vi "Aliases Page.vi"(8 "error in (no error)":errorcluster, 11 "Node Ptr":T4 format="%.0x") -> (0 "error out":errorcluster)   [LabVIEW 2017, in "Routing and Faulting System Explorer.lvlib"]
uses:
  Routing and Faulting System Explorer.lvlib
  <vilib>/NI Veristand/Custom Device API/Custom Device Item Ref.ctl
  Alias.ctl
  Endpoint.ctl
  Shared/UI Common/Sort Button.ctl
  Aliases Page Controls.ctl
  16100924-b29d-4153-bcd0-e39b01036c8d.vi
  16100924-b29d-4153-bcd0-e39b01036c8d.vi/8c7ce3ae-3804-454d-a5c4-51ab498be0b3.vi
  16100924-b29d-4153-bcd0-e39b01036c8d.vi/30b866c3-8f47-4b43-8d37-8753fc540d9b.vi
  <vilib>/NI VeriStand/Custom Device API/Custom Device API.lvlib
  Shared/UI Common/UI Common.lvlib
panel:
  in  "Sort":T1
  out "Alias":string="Alias"
  out "Endpoint":string="Endpoint"
  out "Aliases":T2[](array[typedef])
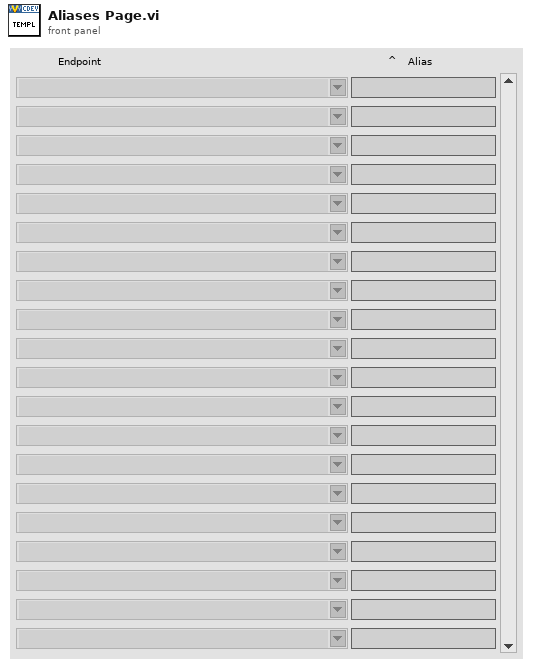
[diagram p1: front panel]
types:
  T1 = typedef "UI Common.lvlib/Sort Button.ctl" = bool
  T2 = typedef "Routing and Faulting System Explorer.lvlib/Alias.ctl" = cluster{"Endpoint":T3, "Alias":string}
  T3 = typedef "Routing and Faulting System Explorer.lvlib/Endpoint.ctl" = string
  T4 = typedef "Custom Device API.lvlib/Custom Device Item Ref.ctl" = u64
  T5 = typedef "Routing and Faulting System Explorer.lvlib/Aliases Page Controls.ctl" = cluster{"Aliases":refnum<vi>, "Endpoint":refnum<vi>, "Alias":refnum<vi>, "Sort":refnum<vi>}
  T6 = typedef "Custom Device API.lvlib/Custom Device Commands.ctl" = enum16{"Default", "Item renamed", "Shutdown", "Dynamic button pressed"}
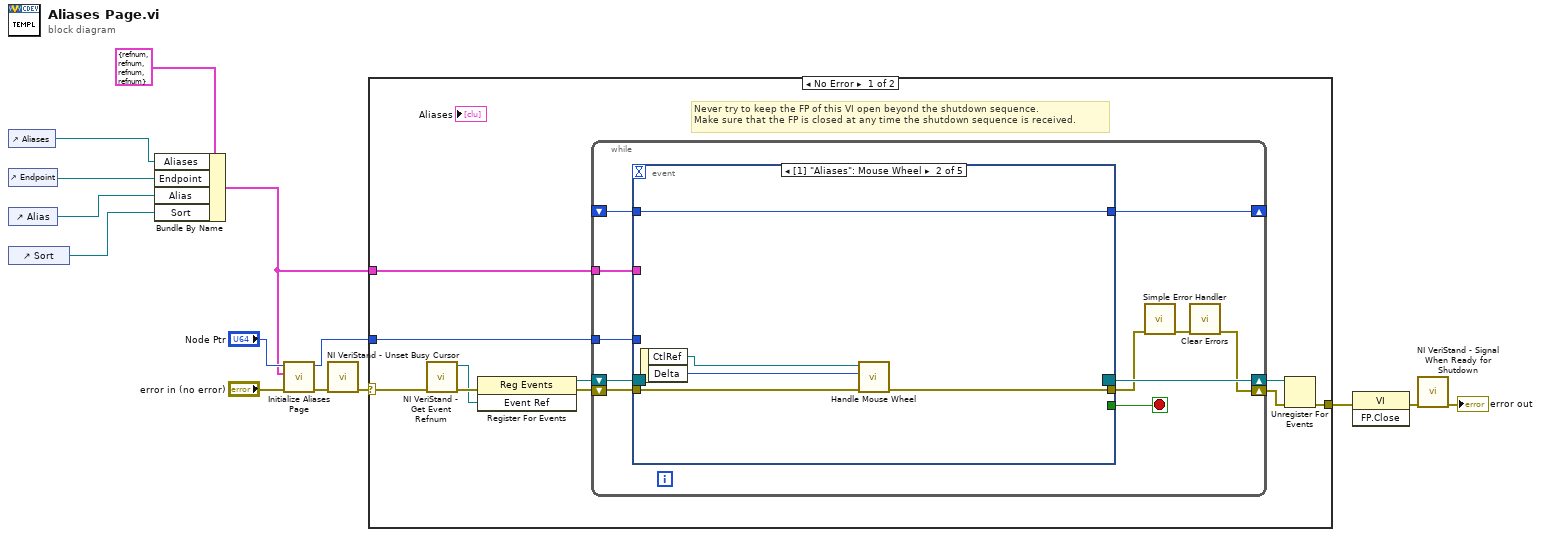
[diagram p0: block diagram]
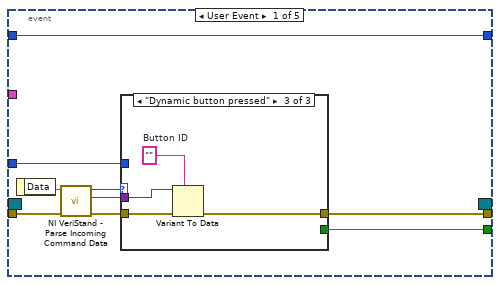
[diagram p2: hidden frame]
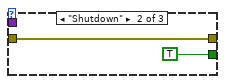
[diagram p4: hidden frame]
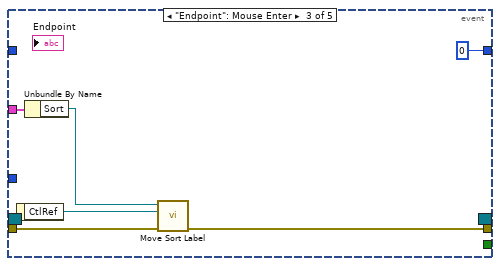
[diagram p5: hidden frame]
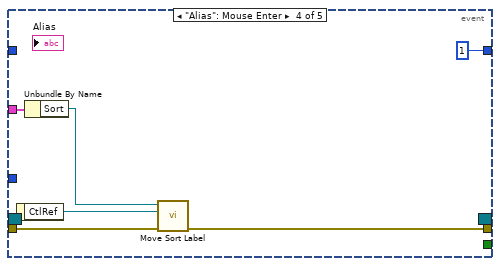
[diagram p6: hidden frame]
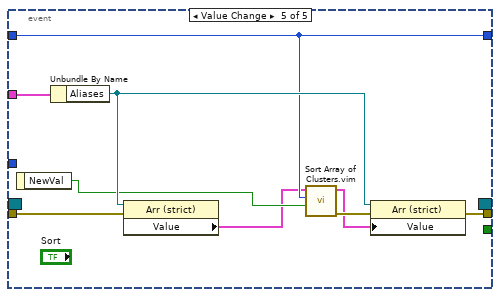
[diagram p7: hidden frame]
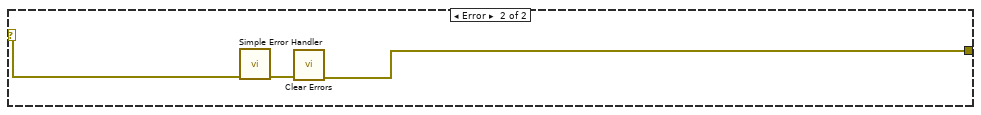
[diagram p8: hidden frame]
diagram:
  n1 = control-ref of="Aliases"() -> (w1:refnum<vi>)
  n2 = control-ref of="Endpoint"() -> (w8:refnum<vi>)
  n3 = control-ref of="Alias"() -> (w7:refnum<vi>)
  n4 = control-ref of="Sort"() -> (w6:refnum<vi>)
  n5 = Bundle By Name(cluster=T5 {"Aliases"=refnum, "Endpoint"=refnum, "Alias"=refnum, "Sort"=refnum} ("Aliases Page Controls"), "Aliases"=w1, "Endpoint"=w8, "Alias"=w7, "Sort"=w6) -> (w2:T5)
  n6 = call "Initialize Aliases Page.vi"("error in (no error)"="error in (no error)", "Aliases Page Controls"=w2, "Aliases Ref in"="Node Ptr") -> ("error out"=w5:errorcluster, "Aliases Ref out"=w9:T4)  [unwired: 7 in]
  n7 = call <vilib>:"NI VeriStand - Unset Busy Cursor.vi"("error in (no error)"=w5) -> ("error out"=w12:errorcluster)  [unwired: 10 out]
  n8 = case shown="No Error" w12 {
    selector: w12 -> [w19 w80]
    tunnel: [w22 w78] -> w14
    tunnel: w9 -> [w20 _]
    tunnel: w2 -> [w17 _]
    frame No Error {
      # "Never try to keep the FP of this VI open beyond the shutdown sequence.\nMake sure that the FP is closed at any time the shutdown sequence is received."
      n9 = call <vilib>:"NI VeriStand - Get Event Refnum.vi"("error in (no error)"=w19) -> ("error out"=w16:errorcluster, "Event Ref"=w15:refnum<user-event>)  [unwired: 9 out]
      n10 = register-events(error in=w16, w15) -> (reference out=w21:refnum<event-registration>, error out=w18:errorcluster)  [unwired: 1 in]
      n11 = while {
        tunnel: w20 -> [w31]
        shift-right: [w28] -> w23
        shift-left: w18 -> [w34]
        shift-right: [w35] -> w24
        shift-left: w21 -> [w33]
        shift-right: [w27] -> _
        shift-left: _ -> [w25]
        tunnel: w17 -> [w26]
        stop <- w32 stop-if-true
        n12 = event shown="[1] \"Aliases\": Mouse Wheel" {
          selector: w33 -> [_ _ _ _ _]
          dyn-events: [_ _ _ _ _] -> w35
          timeout: _ -> [_ _ _ _ _]
          tunnel: w34 -> [w44 w54 w62 w68 w77]
          tunnel: [w40 _ _ _ _] -> w32
          tunnel: [w39 w53 w61 w67 w74] -> w30
          tunnel: w31 -> [w38 _ _ _ _]
          tunnel: [w36 w56 0 ("index of element") 1 ("index of element") w71] -> w27
          tunnel: w26 -> [_ _ w58 w64 w76]
          tunnel: w25 -> [w36 w56 _ _ w71]
          event User Event {
            n13 = event-data() -> ("Data"=w43:string)  [unwired: 1 out]
            n14 = call <vilib>:"NI VeriStand - Parse Incoming Command Data.vi"("error in (no error)"=w44, "Incoming data"=w43) -> ("error out"=w42:errorcluster, "Outgoing data"=w37:variant, "Action"=w41:T6)  [unwired: 7 out]
            n15 = case shown="\"Dynamic button pressed\"" w41 {
              tunnel: w42 -> [w45 w46 w51]
              tunnel: [_ TRUE _] -> w40
              tunnel: [w45 w46 w48] -> w39
              tunnel: w38 -> [_ _ _]
              tunnel: w37 -> [_ _ w50]
              frame "Default", Default {
              }
              frame "Shutdown" {
              }
              frame "Dynamic button pressed" {
                w49 = ""  # Button ID
                n16 = Variant To Data(error in=w51, type=w49, Variant=w50) -> (error out=w48:errorcluster)  [unwired: 1 out]
              }
            }
          }
          event "Aliases": Mouse Wheel {
            n17 = event-data() -> ("CtlRef"=w55:refnum<vi>, "Delta"=w52:i32)  [unwired: 1 out]
            n18 = call "Handle Mouse Wheel.vi"("error in (no error)"=w54, "delta"=w52, "Array Refnum"=w55) -> ("error out"=w53:errorcluster)  [unwired: 7 in, 1 out]
          }
          event "Endpoint": Mouse Enter {
            n19 = event-data() -> ("CtlRef"=w60:refnum<vi>)  [unwired: 1 out]
            n20 = Unbundle By Name(w58) -> ("Sort"=w57:refnum<vi>)
            n21 = call "Move Sort Label.vi"("error in (no error)"=w62, "Target Label"=w60, "Sort"=w57) -> ("error out"=w61:errorcluster)  [unwired: 8 in]
          }
          event "Alias": Mouse Enter {
            n22 = event-data() -> ("CtlRef"=w66:refnum<vi>)  [unwired: 1 out]
            n23 = Unbundle By Name(w64) -> ("Sort"=w63:refnum<vi>)
            n24 = call "Move Sort Label.vi"("error in (no error)"=w68, "Target Label"=w66, "Sort"=w63) -> ("error out"=w67:errorcluster)  [unwired: 8 in]
          }
          event Value Change {
            n25 = event-data() -> ("NewVal"=w72:T1)  [unwired: 1 out]
            n26 = Unbundle By Name(w76) -> ("Aliases"=w73:refnum<vi>)
            n27 = property class="Arr (strict)"(reference=w73, error in=w77) -> ("Value"=w69:T2[])  [unwired: 2 out]
            n28 = call "Sort Array of Clusters.vim"("Descending"=w72, "index"=w71, "Array"=w69) -> ("error out"=w75:errorcluster, "Sorted Array"=w70:T2[])  [unwired: 7 in]
            n29 = property class="Arr (strict)"(reference=w73, error in=w75, "Value"=w70) -> (error out=w74:errorcluster)  [unwired: 1 out]
          }
        }
        n30 = call <vilib>:"Simple Error Handler.vi"("error in (no error)"=w30) -> ("error out"=w29:errorcluster)  [unwired: 1 in, 7 out]
        n31 = call <vilib>:"Clear Errors.vi"("error in (no error)"=w29) -> ("error out"=w28:errorcluster)  [unwired: 1 in, 5 out]
      }
      n32 = Unregister For Events(event registration refnum=w24, error in=w23) -> (error out=w22:errorcluster)
    }
    frame Error {
      n33 = call <vilib>:"Simple Error Handler.vi"("error in (no error)"=w80) -> ("error out"=w79:errorcluster)  [unwired: 1 in, 7 out]
      n34 = call <vilib>:"Clear Errors.vi"("error in (no error)"=w79) -> ("error out"=w78:errorcluster)  [unwired: 1 in, 5 out]
    }
  }
  n35 = invoke class="VI" method="FP.Close"(error in=w14) -> (error out=w4:errorcluster)  [unwired: 2 in, 2 out]
  n36 = call <vilib>:"NI VeriStand - Signal When Ready for Shutdown.vi"("error in (no error)"=w4) -> ("error out"=→"error out":errorcluster)  [unwired: 10 out]
